vi "init_box_1.vi"(0 "Box I VISA Name":refnum<visa-resource-name>, 7 "Controls Cluster":T1, 11 "error in (no error)":errorcluster) -> (4 "Box I VISA Name":refnum<visa-resource-name>, 13 "Trap Delay Array":dbl[](array[numeric]), 15 "error out":errorcluster)   [LabVIEW 2023]
uses:
  <instrlib>/Quantum Composers 9000 Series/Public/Configure/Configure Chan Mode (Normal).vi
  <instrlib>/Quantum Composers 9000 Series/Public/Configure/Configure Sys (To) Mode (Normal).vi
  <instrlib>/Quantum Composers 9000 Series/Public/Action-Status/Query Sys (To) Parameters (Mode).vi
  <instrlib>/Quantum Composers 9000 Series/Quantum Composers 9000 Series.lvlib
panel:
  out "Controls Cluster Out":T1
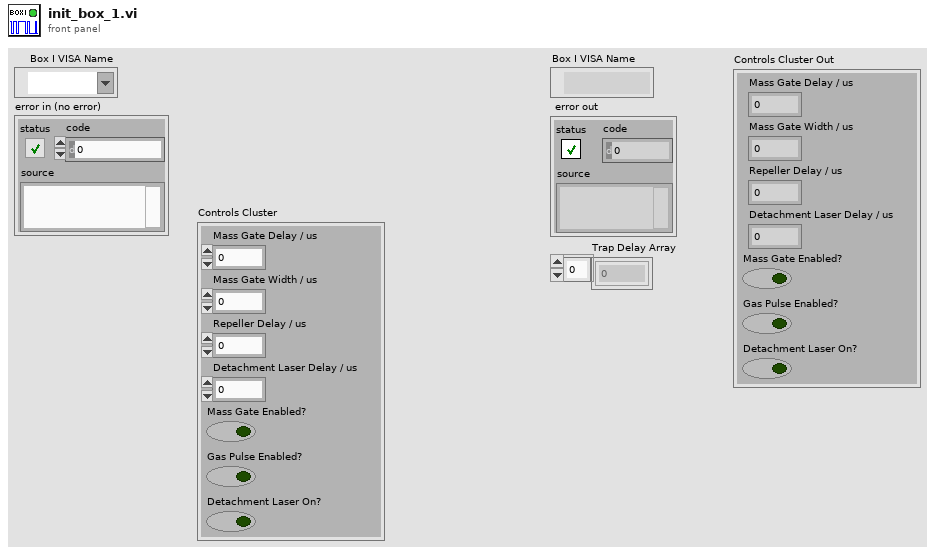
[diagram p1: front panel]
types:
  T1 = cluster{"Mass Gate Delay / us":dbl, "Mass Gate Width / us":dbl, "Repeller Delay / us":dbl, "Detachment Laser Delay / us":dbl, "Mass Gate Enabled?":bool, "Gas Pulse Enabled?":bool, "Detachment Laser On?":bool}
  T2 = enum16{"Disabled", "Pulse Inhibit", "Output Inhibit"}
  T3 = cluster{" Mode":enum16{"Normal", "Single", "Burst", "Duty Cycle"}, "Burst #":i32, "DC Off":i32, "DC On":i32, "Period":dbl}
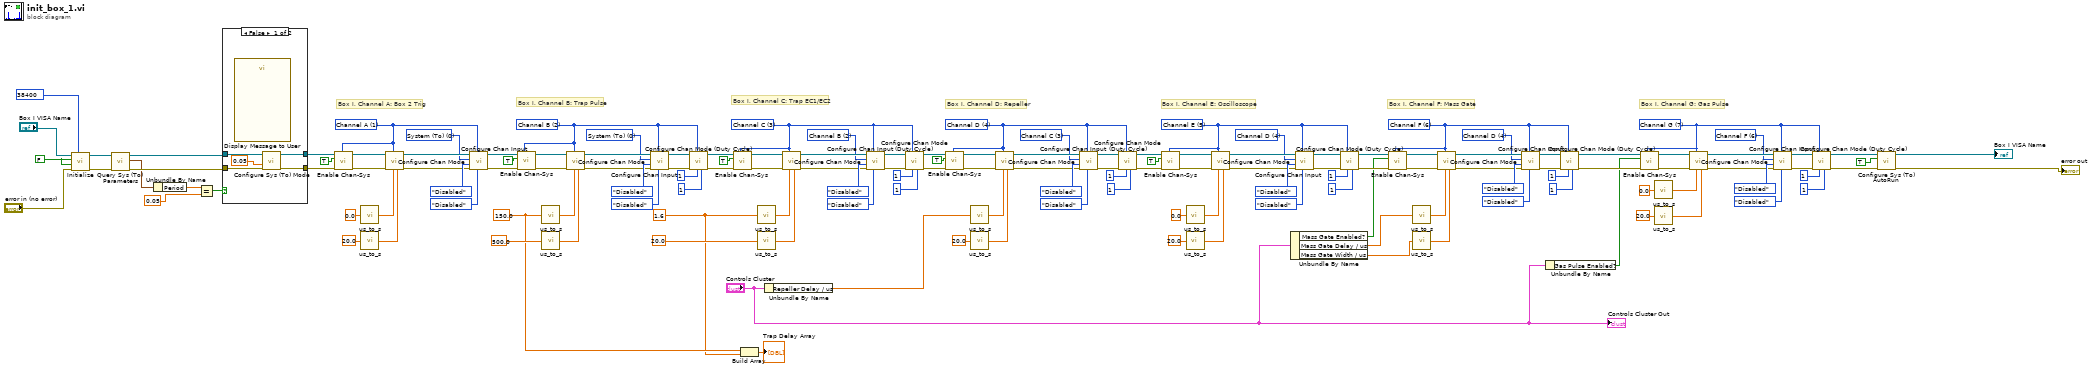
[diagram p0: block diagram]
diagram:
  w16 = u32 38400 items=["4800"=4600, "9600"=9600, "19200"=19200, "38400"=38400, "57600"=57600, "115200"=115200] ("Baud Rate (9600)")
  w31 = FALSE ("ID Query? (T: Yes)")
  w76 = 6 items=["System (To)", "Channel A", "Channel B", "Channel C", "Channel D", "Channel E", "Channel F", "Channel G", "Channel H"] ("Sync Source (0:To)")
  w33 = 7 items=["Channel A"=1, "Channel B"=2, "Channel C"=3, "Channel D"=4, "Channel E"=5, "Channel F"=6, "Channel G"=7, "Channel H"=8] ("Channel (1:Chan A)")
  w89 = 4 items=["System (To)", "Channel A", "Channel B", "Channel C", "Channel D", "Channel E", "Channel F", "Channel G", "Channel H"] ("Sync Source (0:To)")
  w32 = 6 items=["Channel A"=1, "Channel B"=2, "Channel C"=3, "Channel D"=4, "Channel E"=5, "Channel F"=6, "Channel G"=7, "Channel H"=8] ("Channel (1:Chan A)")
  w98 = 4 items=["System (To)", "Channel A", "Channel B", "Channel C", "Channel D", "Channel E", "Channel F", "Channel G", "Channel H"] ("Sync Source (0:To)")
  w40 = 5 items=["Channel A"=1, "Channel B"=2, "Channel C"=3, "Channel D"=4, "Channel E"=5, "Channel F"=6, "Channel G"=7, "Channel H"=8] ("Channel (1:Chan A)")
  w110 = 3 items=["System (To)", "Channel A", "Channel B", "Channel C", "Channel D", "Channel E", "Channel F", "Channel G", "Channel H"] ("Sync Source (0:To)")
  w47 = 4 items=["Channel A"=1, "Channel B"=2, "Channel C"=3, "Channel D"=4, "Channel E"=5, "Channel F"=6, "Channel G"=7, "Channel H"=8] ("Channel (1:Chan A)")
  w122 = 2 items=["System (To)", "Channel A", "Channel B", "Channel C", "Channel D", "Channel E", "Channel F", "Channel G", "Channel H"] ("Sync Source (0:To)")
  w18 = 1.6 ("Time / us")
  w53 = 3 items=["Channel A"=1, "Channel B"=2, "Channel C"=3, "Channel D"=4, "Channel E"=5, "Channel F"=6, "Channel G"=7, "Channel H"=8] ("Channel (1:Chan A)")
  w133 = 0 items=["System (To)", "Channel A", "Channel B", "Channel C", "Channel D", "Channel E", "Channel F", "Channel G", "Channel H"] ("Sync Source (0:To)")
  w19 = 150.0 ("Time / us")
  w59 = 2 items=["Channel A"=1, "Channel B"=2, "Channel C"=3, "Channel D"=4, "Channel E"=5, "Channel F"=6, "Channel G"=7, "Channel H"=8] ("Channel (1:Chan A)")
  w140 = 0 items=["System (To)", "Channel A", "Channel B", "Channel C", "Channel D", "Channel E", "Channel F", "Channel G", "Channel H"] ("Sync Source (0:To)")
  w65 = 1 items=["Channel A"=1, "Channel B"=2, "Channel C"=3, "Channel D"=4, "Channel E"=5, "Channel F"=6, "Channel G"=7, "Channel H"=8] ("Channel (1:Chan A)")
  # "Box I, Channel G: Gas Pulse"
  # "Box I, Channel F: Mass Gate"
  # "Box I, Channel E: Oscilloscope"
  # "Box I, Channel D: Repeller"
  # "Box I, Channel C: Trap EC1/EC2"
  # "Box I, Channel B: Trap Pulse"
  # "Box I, Channel A: Box 2 Trig"
  n1 = call <instrlib>:"Initialize.vi"("Baud Rate (9600)"=w16, "error in (no error)"="error in (no error)", "Reset? (T: Yes)"=w31, "ID Query? (T: Yes)"=w31, "VISA resource name"="Box I VISA Name") -> ("error out"=w9:errorcluster, "VISA resource name out"=w10:refnum<visa-resource-name>)  [unwired: 5 in]
  n2 = call-poly <instrlib>:"Query Sys (To) Parameters.vi"("error in (no error)"=w9, "VISA resource name"=w10) -> ("error out"=w7:errorcluster, "Mode Parameters"=w6:T3, "VISA resource name out"=w8:refnum<visa-resource-name>)  [unwired: 7 in]
  n3 = Unbundle By Name(w6) -> ("Period"=w3:dbl)
  n4 = Equal?(x=w3, y=0.05) -> (x = y?=w1:bool)
  n5 = case shown="False" w1 {
    tunnel: w8 -> [w152 w155]
    tunnel: w7 -> [w151 w154]
    tunnel: [w150 w155] -> w5
    tunnel: [w149 w154] -> w4
    frame False {
      n6 = call "Display Message to User"() -> ()  [unwired: 10 in, 2 out]
      n7 = call-poly <instrlib>:"Configure Sys (To) Mode.vi"("error in (no error)"=w151, "Period (100 msec)"=0.05, "VISA resource name"=w152) -> ("error out"=w149:errorcluster, "VISA resource name out"=w150:refnum<visa-resource-name>)  [unwired: 7 in]
    }
    frame True {
    }
  }
  n8 = call <instrlib>:"Enable Chan-Sys.vi"("Channel (1:Chan A)"=w65, "error in (no error)"=w4, "State (T:Enabled)"=TRUE, "VISA resource name"=w5) -> ("error out"=w66:errorcluster, "VISA resource name out"=w67:refnum<visa-resource-name>)  [unwired: 6 in]
  n9 = call "us_to_s.vi"("Time / us"=0.0) -> ("Time / s"=w144:dbl)
  n10 = call "us_to_s.vi"("Time / us"=20.0) -> ("Time / s"=w143:dbl)
  n11 = call-poly <instrlib>:"Configure Chan Mode.vi"("Width (10 msec)"=w143, "Delay (10 msec)"=w144, "Channel (1:Chan A)"=w65, "error in (no error)"=w66, "VISA resource name"=w67) -> ("error out"=w145:errorcluster, "VISA resource name out"=w146:refnum<visa-resource-name>)  [unwired: 5 in]
  n12 = call <instrlib>:"Configure Chan Input.vi"("Gate Mode (0:Disabled)"=T2."Disabled", "Channel (1:Chan A)"=w65, "error in (no error)"=w145, "Gate Logic (0:Disabled)"=enum16{"Disabled", "Low", "High"}."Disabled", "Sync Source (0:To)"=w140, "VISA resource name"=w146) -> ("error out"=w60:errorcluster, "VISA resource name out"=w61:refnum<visa-resource-name>)  [unwired: 4 in]
  n13 = call <instrlib>:"Enable Chan-Sys.vi"("Channel (1:Chan A)"=w59, "error in (no error)"=w60, "State (T:Enabled)"=TRUE, "VISA resource name"=w61) -> ("error out"=w62:errorcluster, "VISA resource name out"=w63:refnum<visa-resource-name>)  [unwired: 6 in]
  n14 = call "us_to_s.vi"("Time / us"=w19) -> ("Time / s"=w22:dbl)
  n15 = call "us_to_s.vi"("Time / us"=500.0) -> ("Time / s"=w135:dbl)
  n16 = call-poly <instrlib>:"Configure Chan Mode.vi"("Width (10 msec)"=w135, "Delay (10 msec)"=w22, "Channel (1:Chan A)"=w59, "error in (no error)"=w62, "VISA resource name"=w63) -> ("error out"=w136:errorcluster, "VISA resource name out"=w137:refnum<visa-resource-name>)  [unwired: 5 in]
  n17 = call <instrlib>:"Configure Chan Input.vi"("Gate Mode (0:Disabled)"=T2."Disabled", "Channel (1:Chan A)"=w59, "error in (no error)"=w136, "Gate Logic (0:Disabled)"=enum16{"Disabled", "Low", "High"}."Disabled", "Sync Source (0:To)"=w133, "VISA resource name"=w137) -> ("error out"=w131:errorcluster, "VISA resource name out"=w132:refnum<visa-resource-name>)  [unwired: 4 in]
  n18 = call <instrlib>:"Configure Chan Mode (Duty Cycle).vi"("Chan DC Off (10)"=1, "Chan DC On (10)"=1, "Channel (1:Chan A)"=w59, "error in (no error)"=w131, "VISA resource name"=w132) -> ("error out"=w54:errorcluster, "VISA resource name out"=w55:refnum<visa-resource-name>)  [unwired: 5 in]
  n19 = call <instrlib>:"Enable Chan-Sys.vi"("Channel (1:Chan A)"=w53, "error in (no error)"=w54, "State (T:Enabled)"=TRUE, "VISA resource name"=w55) -> ("error out"=w56:errorcluster, "VISA resource name out"=w57:refnum<visa-resource-name>)  [unwired: 6 in]
  n20 = Build Array(w19, w18) -> (→"Trap Delay Array":dbl[])
  n21 = call "us_to_s.vi"("Time / us"=w18) -> ("Time / s"=w21:dbl)
  n22 = call "us_to_s.vi"("Time / us"=20.0) -> ("Time / s"=w124:dbl)
  n23 = Unbundle By Name("Controls Cluster") -> ("Repeller Delay / us"=w20:dbl)
  n24 = call-poly <instrlib>:"Configure Chan Mode.vi"("Width (10 msec)"=w124, "Delay (10 msec)"=w21, "Channel (1:Chan A)"=w53, "error in (no error)"=w56, "VISA resource name"=w57) -> ("error out"=w125:errorcluster, "VISA resource name out"=w126:refnum<visa-resource-name>)  [unwired: 5 in]
  n25 = call <instrlib>:"Configure Chan Input.vi"("Gate Mode (0:Disabled)"=T2."Disabled", "Channel (1:Chan A)"=w53, "error in (no error)"=w125, "Gate Logic (0:Disabled)"=enum16{"Disabled", "Low", "High"}."Disabled", "Sync Source (0:To)"=w122, "VISA resource name"=w126) -> ("error out"=w120:errorcluster, "VISA resource name out"=w121:refnum<visa-resource-name>)  [unwired: 4 in]
  n26 = call <instrlib>:"Configure Chan Mode (Duty Cycle).vi"("Chan DC Off (10)"=1, "Chan DC On (10)"=1, "Channel (1:Chan A)"=w53, "error in (no error)"=w120, "VISA resource name"=w121) -> ("error out"=w48:errorcluster, "VISA resource name out"=w49:refnum<visa-resource-name>)  [unwired: 5 in]
  n27 = call <instrlib>:"Enable Chan-Sys.vi"("Channel (1:Chan A)"=w47, "error in (no error)"=w48, "State (T:Enabled)"=TRUE, "VISA resource name"=w49) -> ("error out"=w50:errorcluster, "VISA resource name out"=w51:refnum<visa-resource-name>)  [unwired: 6 in]
  n28 = call "us_to_s.vi"("Time / us"=w20) -> ("Time / s"=w113:dbl)
  n29 = call "us_to_s.vi"("Time / us"=20.0) -> ("Time / s"=w112:dbl)
  n30 = call-poly <instrlib>:"Configure Chan Mode.vi"("Width (10 msec)"=w112, "Delay (10 msec)"=w113, "Channel (1:Chan A)"=w47, "error in (no error)"=w50, "VISA resource name"=w51) -> ("error out"=w114:errorcluster, "VISA resource name out"=w115:refnum<visa-resource-name>)  [unwired: 5 in]
  n31 = call <instrlib>:"Configure Chan Input.vi"("Gate Mode (0:Disabled)"=T2."Disabled", "Channel (1:Chan A)"=w47, "error in (no error)"=w114, "Gate Logic (0:Disabled)"=enum16{"Disabled", "Low", "High"}."Disabled", "Sync Source (0:To)"=w110, "VISA resource name"=w115) -> ("error out"=w108:errorcluster, "VISA resource name out"=w109:refnum<visa-resource-name>)  [unwired: 4 in]
  n32 = call <instrlib>:"Configure Chan Mode (Duty Cycle).vi"("Chan DC Off (10)"=1, "Chan DC On (10)"=1, "Channel (1:Chan A)"=w47, "error in (no error)"=w108, "VISA resource name"=w109) -> ("error out"=w42:errorcluster, "VISA resource name out"=w43:refnum<visa-resource-name>)  [unwired: 5 in]
  n33 = call <instrlib>:"Enable Chan-Sys.vi"("Channel (1:Chan A)"=w40, "error in (no error)"=w42, "State (T:Enabled)"=TRUE, "VISA resource name"=w43) -> ("error out"=w44:errorcluster, "VISA resource name out"=w45:refnum<visa-resource-name>)  [unwired: 6 in]
  n34 = call "us_to_s.vi"("Time / us"=0.0) -> ("Time / s"=w101:dbl)
  n35 = call "us_to_s.vi"("Time / us"=20.0) -> ("Time / s"=w100:dbl)
  n36 = call-poly <instrlib>:"Configure Chan Mode.vi"("Width (10 msec)"=w100, "Delay (10 msec)"=w101, "Channel (1:Chan A)"=w40, "error in (no error)"=w44, "VISA resource name"=w45) -> ("error out"=w102:errorcluster, "VISA resource name out"=w103:refnum<visa-resource-name>)  [unwired: 5 in]
  n37 = Unbundle By Name("Controls Cluster") -> ("Mass Gate Enabled?"=w28:bool, "Mass Gate Delay / us"=w27:dbl, "Mass Gate Width / us"=w26:dbl)
  n38 = call <instrlib>:"Configure Chan Input.vi"("Gate Mode (0:Disabled)"=T2."Disabled", "Channel (1:Chan A)"=w40, "error in (no error)"=w102, "Gate Logic (0:Disabled)"=enum16{"Disabled", "Low", "High"}."Disabled", "Sync Source (0:To)"=w98, "VISA resource name"=w103) -> ("error out"=w96:errorcluster, "VISA resource name out"=w97:refnum<visa-resource-name>)  [unwired: 4 in]
  n39 = call <instrlib>:"Configure Chan Mode (Duty Cycle).vi"("Chan DC Off (10)"=1, "Chan DC On (10)"=1, "Channel (1:Chan A)"=w40, "error in (no error)"=w96, "VISA resource name"=w97) -> ("error out"=w38:errorcluster, "VISA resource name out"=w39:refnum<visa-resource-name>)  [unwired: 5 in]
  n40 = call <instrlib>:"Enable Chan-Sys.vi"("Channel (1:Chan A)"=w32, "error in (no error)"=w38, "State (T:Enabled)"=w28, "VISA resource name"=w39) -> ("error out"=w36:errorcluster, "VISA resource name out"=w37:refnum<visa-resource-name>)  [unwired: 6 in]
  n41 = call "us_to_s.vi"("Time / us"=w27) -> ("Time / s"=w83:dbl)
  n42 = call "us_to_s.vi"("Time / us"=w26) -> ("Time / s"=w82:dbl)
  n43 = call-poly <instrlib>:"Configure Chan Mode.vi"("Width (10 msec)"=w82, "Delay (10 msec)"=w83, "Channel (1:Chan A)"=w32, "error in (no error)"=w36, "VISA resource name"=w37) -> ("error out"=w90:errorcluster, "VISA resource name out"=w91:refnum<visa-resource-name>)  [unwired: 5 in]
  n44 = call <instrlib>:"Configure Chan Input.vi"("Gate Mode (0:Disabled)"=T2."Disabled", "Channel (1:Chan A)"=w32, "error in (no error)"=w90, "Gate Logic (0:Disabled)"=enum16{"Disabled", "Low", "High"}."Disabled", "Sync Source (0:To)"=w89, "VISA resource name"=w91) -> ("error out"=w87:errorcluster, "VISA resource name out"=w88:refnum<visa-resource-name>)  [unwired: 4 in]
  n45 = Unbundle By Name("Controls Cluster") -> ("Gas Pulse Enabled?"=w24:bool)
  n46 = call <instrlib>:"Configure Chan Mode (Duty Cycle).vi"("Chan DC Off (10)"=1, "Chan DC On (10)"=1, "Channel (1:Chan A)"=w32, "error in (no error)"=w87, "VISA resource name"=w88) -> ("error out"=w29:errorcluster, "VISA resource name out"=w30:refnum<visa-resource-name>)  [unwired: 5 in]
  n47 = call <instrlib>:"Enable Chan-Sys.vi"("Channel (1:Chan A)"=w33, "error in (no error)"=w29, "State (T:Enabled)"=w24, "VISA resource name"=w30) -> ("error out"=w34:errorcluster, "VISA resource name out"=w35:refnum<visa-resource-name>)  [unwired: 6 in]
  n48 = call "us_to_s.vi"("Time / us"=0.0) -> ("Time / s"=w71:dbl)
  n49 = call "us_to_s.vi"("Time / us"=20.0) -> ("Time / s"=w70:dbl)
  n50 = call-poly <instrlib>:"Configure Chan Mode.vi"("Width (10 msec)"=w70, "Delay (10 msec)"=w71, "Channel (1:Chan A)"=w33, "error in (no error)"=w34, "VISA resource name"=w35) -> ("error out"=w77:errorcluster, "VISA resource name out"=w78:refnum<visa-resource-name>)  [unwired: 5 in]
  n51 = call <instrlib>:"Configure Chan Input.vi"("Gate Mode (0:Disabled)"=T2."Disabled", "Channel (1:Chan A)"=w33, "error in (no error)"=w77, "Gate Logic (0:Disabled)"=enum16{"Disabled", "Low", "High"}."Disabled", "Sync Source (0:To)"=w76, "VISA resource name"=w78) -> ("error out"=w74:errorcluster, "VISA resource name out"=w75:refnum<visa-resource-name>)  [unwired: 4 in]
  n52 = call <instrlib>:"Configure Chan Mode (Duty Cycle).vi"("Chan DC Off (10)"=1, "Chan DC On (10)"=1, "Channel (1:Chan A)"=w33, "error in (no error)"=w74, "VISA resource name"=w75) -> ("error out"=w14:errorcluster, "VISA resource name out"=w15:refnum<visa-resource-name>)  [unwired: 5 in]
  n53 = call <instrlib>:"Configure Sys (To) AutoRun.vi"("error in (no error)"=w14, "AutoRun (F:Disabled)"=TRUE, "VISA resource name"=w15) -> ("error out"=→"error out":errorcluster, "VISA resource name out"=→"Box I VISA Name":refnum<visa-resource-name>)  [unwired: 7 in]
  "Controls Cluster Out" <- "Controls Cluster"
